vi "Data Check.vi"(9 "Offset In":sgl[](array[numeric]), 11 "X In":sgl[](array[numeric])) -> (0 "error":i32, 1 "Offset Out":sgl[](array[numeric]), 3 "X Out":sgl[](array[numeric]))   [LabVIEW 2017, in "3D Pie Datatype.lvclass"]
uses:
  <vilib>/Math Plots/3D Math Plots/3D Pie/3D Pie Datatype/3D Pie Datatype.lvclass
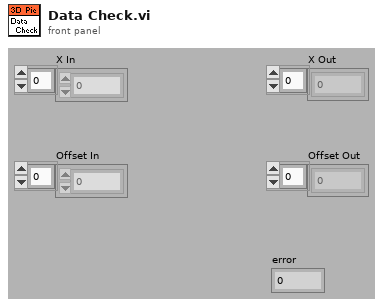
[diagram p1: front panel]
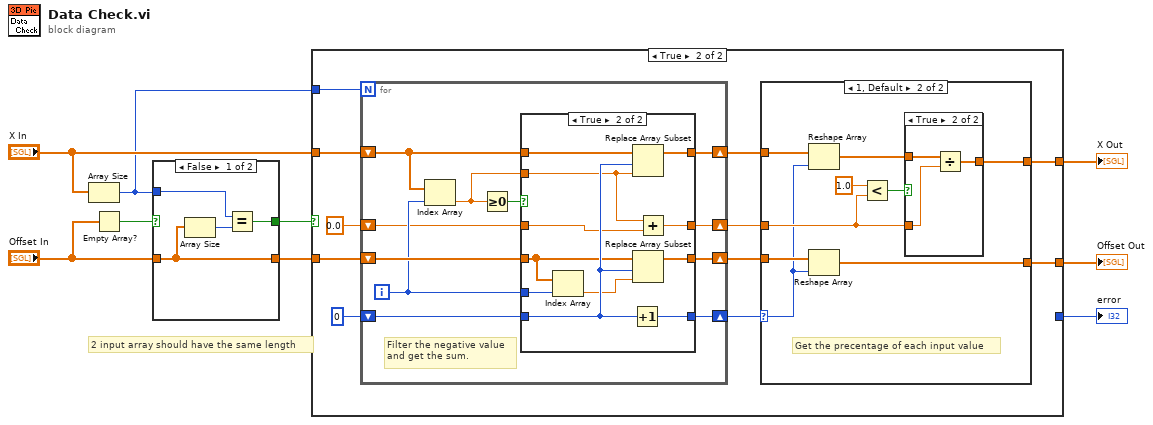
[diagram p0: block diagram]
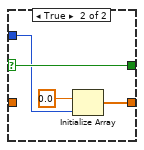
[diagram p2: hidden frame]
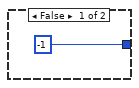
[diagram p3: hidden frame]
diagram:
  # "2 input array should have the same length"
  n1 = Array Size(array="X In") -> (size(s)=w7:i32)
  n2 = Empty Array?(array="Offset In") -> (empty?=w3:bool)
  n3 = case shown="False" w3 {
    selector: w3 -> [_ w17]
    tunnel: [w12 w17] -> w9
    tunnel: w7 -> [w11 w15]
    tunnel: "Offset In" -> [w10 _]
    tunnel: [w10 w16] -> w1
    frame False {
      n4 = Array Size(array=w10) -> (size(s)=w13:i32)
      n5 = Equal?(x=w11, y=w13) -> (x = y?=w12:bool)
    }
    frame True {
      n6 = Initialize Array(sgl 0.0 ("element"), w15) -> (w16:sgl[])
    }
  }
  n7 = case shown="True" w9 {
    tunnel: "X In" -> [_ w29]
    tunnel: w7 -> [_ w28]
    tunnel: [_ w21] -> w6
    tunnel: [_ w20] -> w5
    tunnel: [-1 _] -> w4
    tunnel: w1 -> [_ w19]
    frame False {
    }
    frame True {
      n8 = for {
        N: w28 -> [_]
        shift-right: [w43] -> w24
        shift-left: w29 -> [w52]
        shift-right: [w48] -> w23
        shift-left: w19 -> [w49]
        shift-right: [w47] -> w25
        shift-left: 0 -> [w51]
        shift-right: [w44] -> w22
        shift-left: sgl 0.0 -> [w45]
        i -> [w46]
        # "Filter the negative value \nand get the sum."
        n9 = Index Array(array=w52, index=w46) -> (element=w50:sgl)
        n10 = Greater Or Equal To 0?(x=w50) -> (x >= 0?=w53:bool)
        n11 = case shown="True" w53 {
          tunnel: w52 -> [w57 w68]
          tunnel: w51 -> [w54 w66]
          tunnel: w50 -> [_ w60]
          tunnel: w49 -> [w55 w64]
          tunnel: [w55 w67] -> w48
          tunnel: [w54 w63] -> w47
          tunnel: w46 -> [_ w62]
          tunnel: w45 -> [w56 w61]
          tunnel: [w56 w59] -> w44
          tunnel: [w57 w58] -> w43
          frame False {
          }
          frame True {
            n12 = Index Array(array=w64, index=w62) -> (element=w65:sgl)
            n13 = Increment(x=w66) -> (x+1=w63:i32)
            n14 = Replace Array Subset(array=w68, new element=w60, index=w66) -> (w58:sgl[])
            n15 = Replace Array Subset(array=w64, new element=w65, index=w66) -> (w67:sgl[])
            n16 = Add(x=w60, y=w61) -> (x+y=w59:sgl)
          }
        }
      }
      n17 = case shown="1, Default" w25 {
        selector: w25 -> [_ w33]
        tunnel: w24 -> [_ w31]
        tunnel: w23 -> [_ w34]
        tunnel: w22 -> [_ w36]
        tunnel: [_ w35] -> w21
        tunnel: [_ w32] -> w20
        frame 0 {
        }
        frame 1, Default {
          # "Get the precentage of each input value"
          n18 = Reshape Array(w31, w33) -> (w30:sgl[])
          n19 = Reshape Array(w34, w33) -> (w32:sgl[])
          n20 = Less?(x=sgl 1.0 ("y"), y=w36) -> (x < y?=w38:bool)
          n21 = case shown="True" w38 {
            tunnel: w30 -> [w39 w42]
            tunnel: w36 -> [_ w41]
            tunnel: [w39 w40] -> w35
            frame False {
            }
            frame True {
              n22 = Divide(x=w42, y=w41) -> (x/y=w40:sgl[])
            }
          }
        }
      }
    }
  }
  "X Out" <- w6
  "Offset Out" <- w5
  "error" <- w4
